vi "Get_Coeff_Fr_String.vi"(4 "String Name":string, 5 "Take New Data?":bool, 6 "Prefix":string, 7 "Show Dialog?":bool=TRUE, 8 "Sub String":string, 9 "Inst type":T1=enum."Raw voltage", 10 "Whole String":string) -> (0 "Coefficients Found?":bool, 2 "Calib Constants":dbl[](array[numeric]))   [LabVIEW 2014]
uses:
  Controls/Pressure_Units.ctl
  Controls/Inst_type.ctl
panel:
  in  "Pressure Units":T2
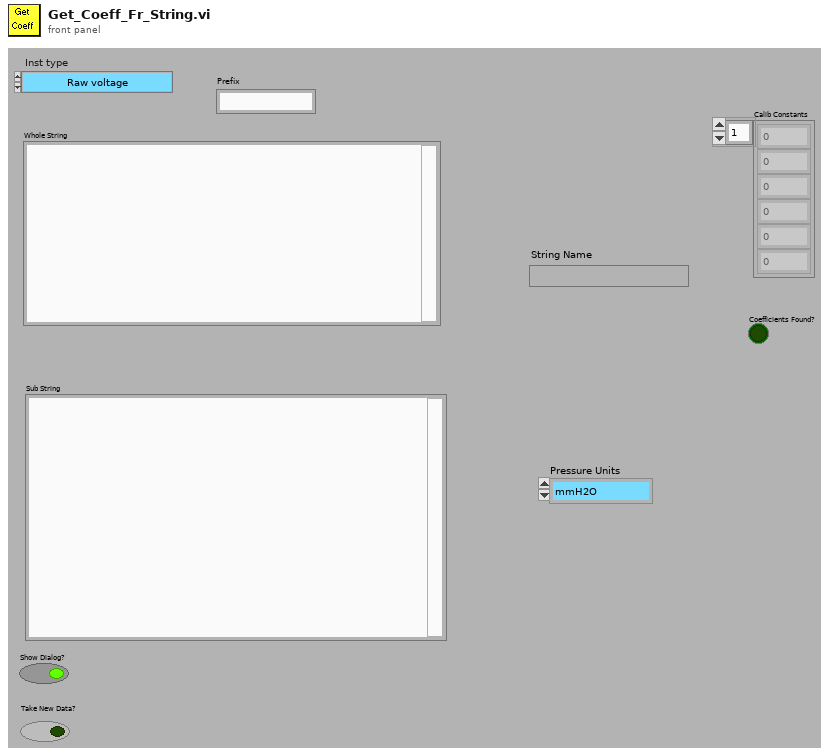
[diagram p1: front panel]
types:
  T1 = typedef "Inst_type.ctl" = enum16{"Propeller anemometer", "Raw voltage", "Pressure Transducer", "Pitot-static tube", "Preston tube", "Hot wire", "Cross wire 1", "Cross wire 2", "Generic Linear", "Generic Polynomial", "Generic BackPoly", "Fast FID", "Thermocouple", "Cold wire", "Pulsed Wire", "LDA Vel", "LDA Tran time", "LDA Arr time", "Microphone"}
  T2 = typedef "Pressure_Units.ctl" = enum16{"mmH2O", "mmHg", "Pa (N/m^2)", "mbar", "bar"}
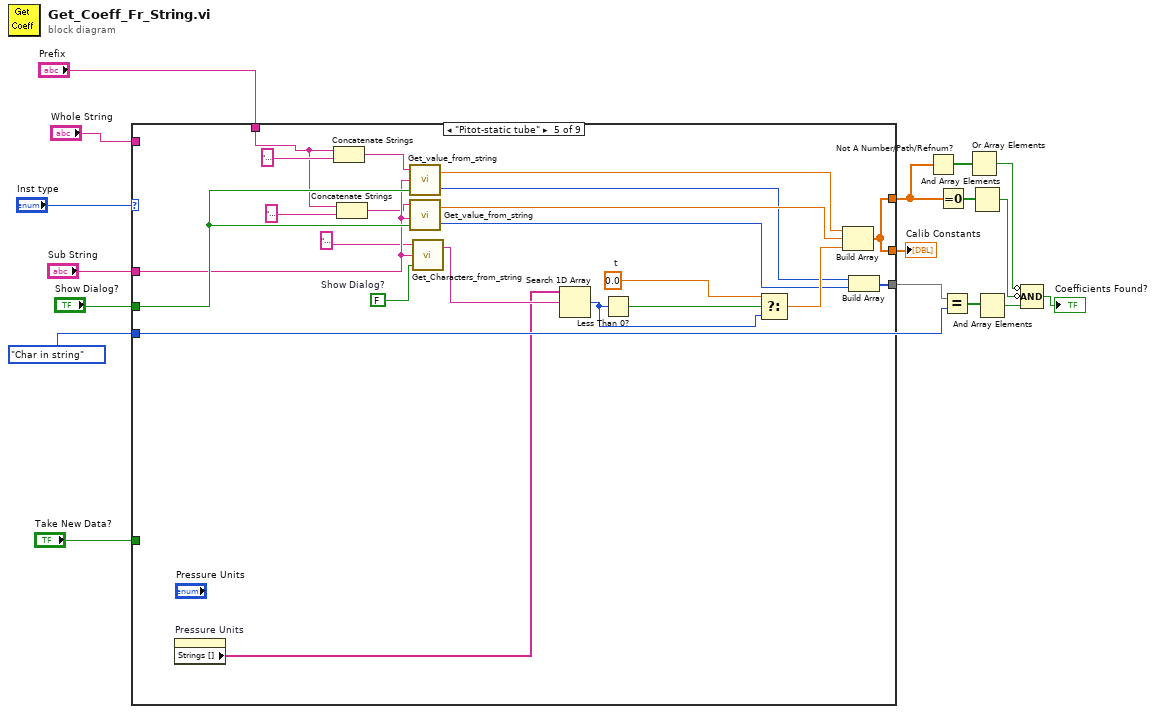
[diagram p0: block diagram]
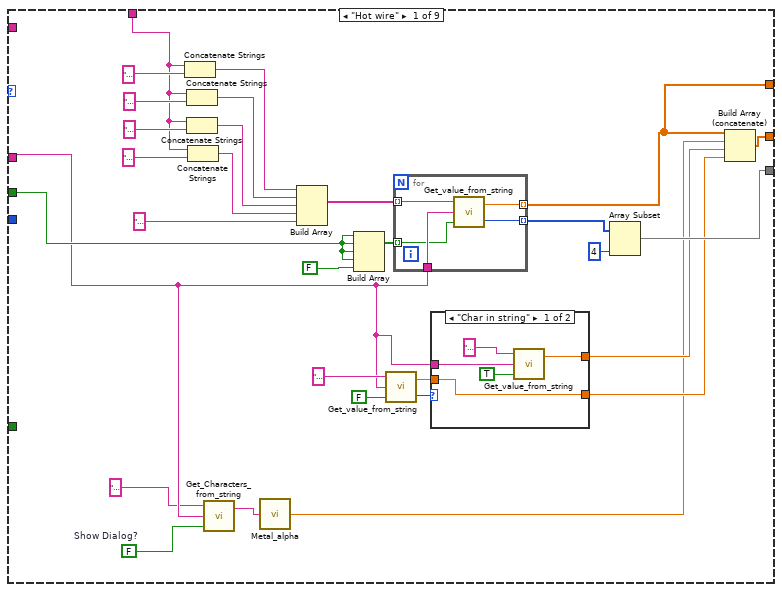
[diagram p2: hidden frame]
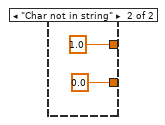
[diagram p3: hidden frame]
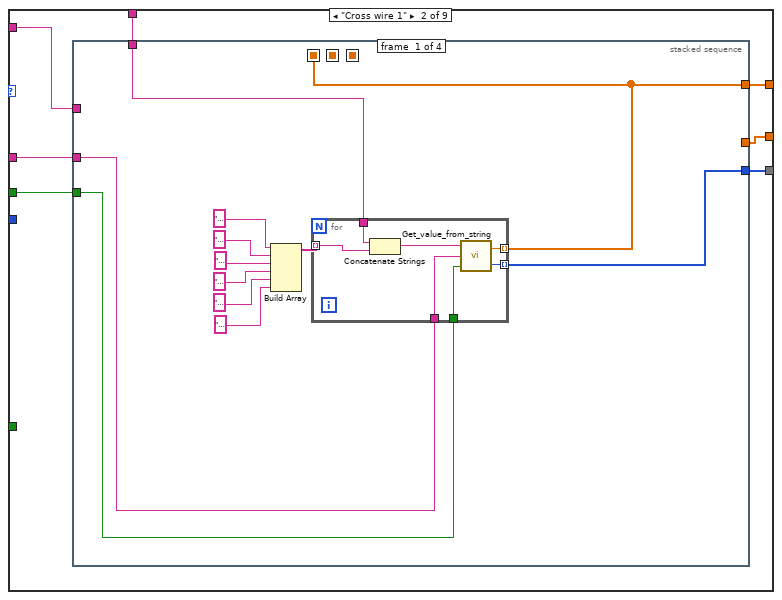
[diagram p4: hidden frame]
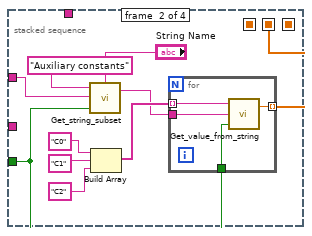
[diagram p5: hidden frame]
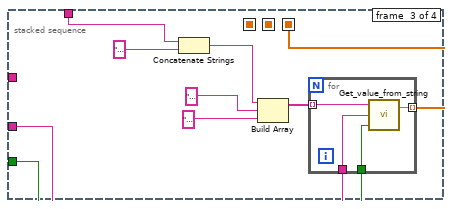
[diagram p6: hidden frame]
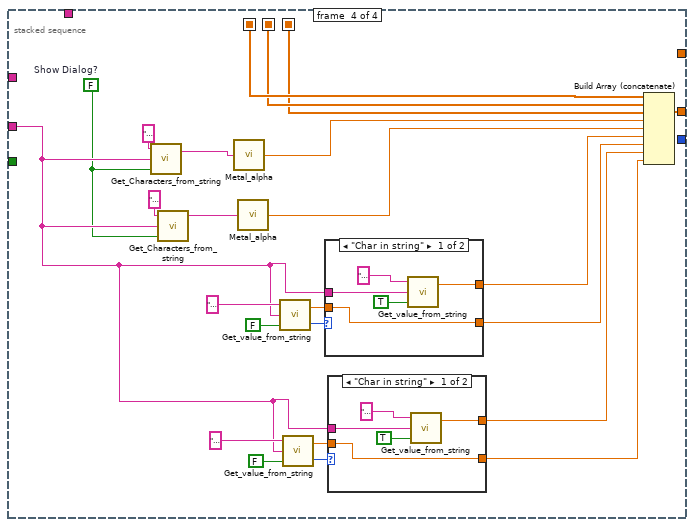
[diagram p7: hidden frame]
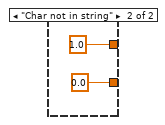
[diagram p8: hidden frame]
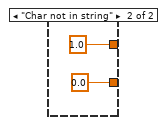
[diagram p9: hidden frame]
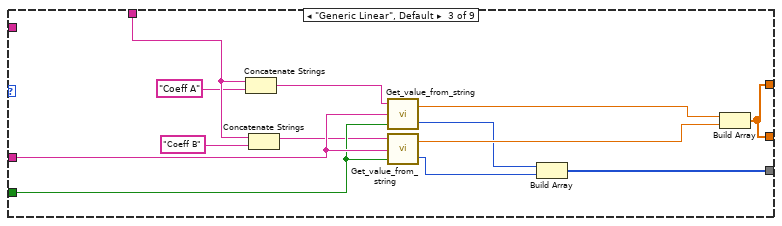
[diagram p10: hidden frame]
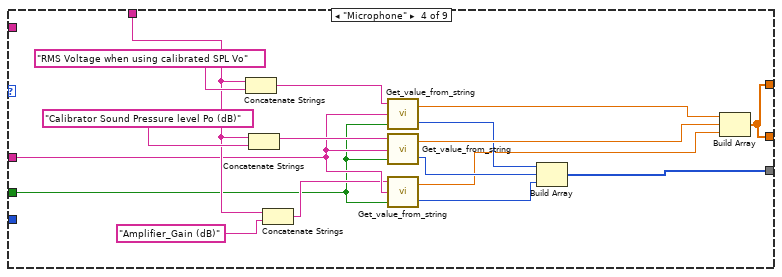
[diagram p11: hidden frame]
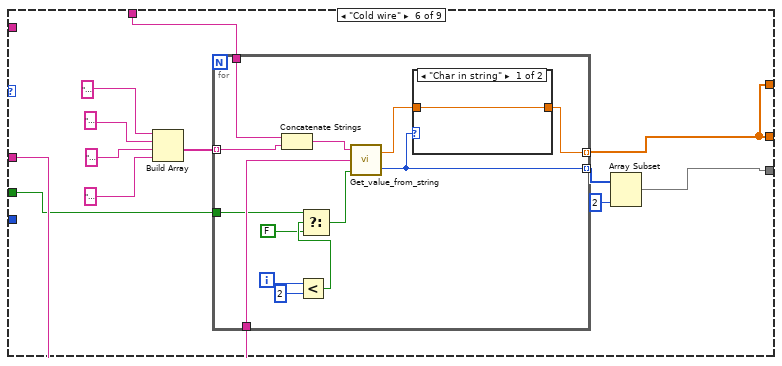
[diagram p12: hidden frame]
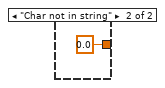
[diagram p13: hidden frame]
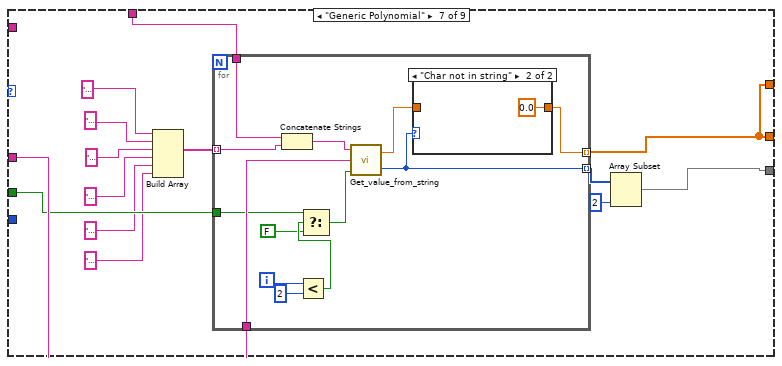
[diagram p14: hidden frame]
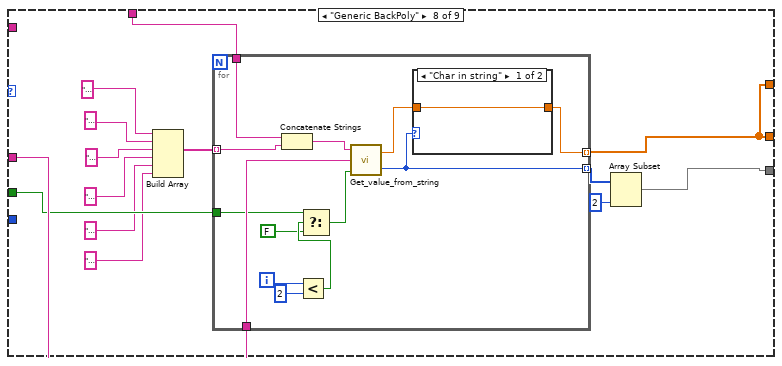
[diagram p16: hidden frame]
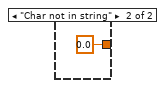
[diagram p17: hidden frame]
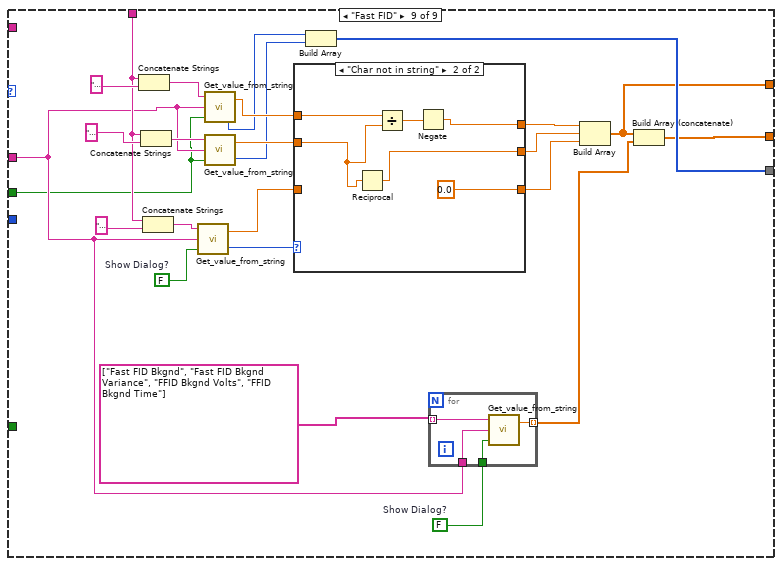
[diagram p18: hidden frame]
diagram:
  w8 = enum16{"Char in string", "Char not in string"}."Char in string" ("Status")
  n1 = case shown="\"Pitot-static tube\"" "Inst type" {
    tunnel: [w47 w66 w151 w171 w181 w202 w231 w260 w288] -> w14
    tunnel: "Sub String" -> [w25 w64 w161 w169 w198 w208 w237 w266 w302]
    tunnel: "Whole String" -> [_ w65 _ _ _ _ _ _ _]
    tunnel: "Show Dialog?" -> [w29 w63 w160 w167 w199 w206 w235 w264 w291]
    tunnel: "Prefix" -> [w37 w62 w159 w170 w184 w207 w236 w265 w305]
    tunnel: "Take New Data?" -> [_ _ _ _ _ _ _ _ _]
    tunnel: [w30 w61 w152 w172 w187 w203 w232 w261 w292] -> w10
    tunnel: w8 -> [_ _ _ _ _ _ _ _ _]
    tunnel: [w21 w60 w151 w171 w181 w202 w231 w260 w287] -> w3
    frame "Hot wire" {
      w44 = FALSE  # Show Dialog?
      n2 = Concatenate Strings(w37, "Coeff A") -> (w33:string)
      n3 = Concatenate Strings(w37, "Coeff B") -> (w34:string)
      n4 = Concatenate Strings(w37, "Coeff n") -> (w35:string)
      n5 = Concatenate Strings(w37, "Calib temp") -> (w36:string)
      n6 = call "Get_Characters_from_string.vi"("Show Dialog?"=w44, "Input string"=w25, "Variable name"="Metal_Type 1") -> ("Value"=w19:string)  [unwired: 1 out]
      n7 = call "Metal_alpha.vi"("Metal_Type"=w19) -> ("alpha (/K)"=w18:dbl)
      n8 = Build Array(w33, w34, w35, w36, "Overheat ratio 1") -> (w45:string[])
      n9 = Build Array(w29, w29, w29, w29, FALSE ("Input Element")) -> (w42:bool[])
      n10 = call "Get_value_from_string.vi"("Show Dialog?"=FALSE, "Input string"=w25, "Variable name"="Offset Voltage 1") -> ("Status"=w26:enum16{"Char in string", "Char not in string"}, "Value"=w23:dbl)
      n11 = for {
        tunnel: w45 -> [w59] mode=indexing
        tunnel: w25 -> [w58]
        tunnel: [w57] -> w21 mode=indexing
        tunnel: w42 -> [w56] mode=indexing
        tunnel: [w55] -> w32 mode=indexing
        n12 = call "Get_value_from_string.vi"("Show Dialog?"=w56, "Input string"=w58, "Variable name"=w59) -> ("Status"=w55:enum16{"Char in string", "Char not in string"}, "Value"=w57:dbl)
      }
      n13 = case shown="\"Char in string\"" w26 {
        tunnel: w25 -> [w52 _]
        tunnel: [w49 1.0 ("Value")] -> w24
        tunnel: w23 -> [w48 _]
        tunnel: [w48 0.0 ("Value")] -> w22
        frame "Char in string" {
          n14 = call "Get_value_from_string.vi"("Show Dialog?"=TRUE, "Input string"=w52, "Variable name"="Gain 1") -> ("Value"=w49:dbl)  [unwired: 1 out]
        }
        frame "Char not in string" {
        }
      }
      n15 = Array Subset(array=w32, length=4) -> (w30:enum16{"Char in string", "Char not in string"}[])  [unwired: 1 in]
      n16 = Build Array (concatenate)(w21, w18, w24, w22) -> (w47:dbl[])
    }
    frame "Cross wire 1" {
      n17 = stacked-sequence {
        seq-local: [w67 _ _ _] -> [_ _ _ w133]
        seq-local: [_ w88 _ _] -> [_ _ _ w132]
        seq-local: [_ _ w105 _] -> [_ _ _ w131]
        tunnel: [_ _ _ w136] -> w66
        tunnel: w65 -> [_ w94 _ _]
        tunnel: w64 -> [w71 _ w107 w122]
        tunnel: w63 -> [w70 w87 w106 _]
        tunnel: w62 -> [w69 _ w100 _]
        tunnel: [w68 _ _ _] -> w61
        tunnel: [w67 _ _ _] -> w60
        frame #0 {
          n18 = Build Array("Coeff A1", "Coeff B1", "Coeff n1", "Coeff A2", "Coeff B2", "Coeff n2") -> (w72:string[])
          n19 = for {
            tunnel: w72 -> [w82] mode=indexing
            tunnel: w71 -> [w85]
            tunnel: [w84] -> w67 mode=indexing
            tunnel: w70 -> [w83]
            tunnel: w69 -> [w80]
            tunnel: [w79] -> w68 mode=indexing
            n20 = Concatenate Strings(w80, w82) -> (w81:string)
            n21 = call "Get_value_from_string.vi"("Show Dialog?"=w83, "Input string"=w85, "Variable name"=w81) -> ("Status"=w79:enum16{"Char in string", "Char not in string"}, "Value"=w84:dbl)
          }
        }
        frame #1 {
          n22 = call "Get_string_subset.vi"("String Name"="String Name", "Show Dialog?"=w87, "String to split"=w94, "File Label"="Auxiliary constants") -> ("Output string"=w89:string)  [unwired: 1 out]
          n23 = Build Array("C0", "C1", "C2") -> (w90:string[])
          n24 = for {
            tunnel: w90 -> [w99] mode=indexing
            tunnel: [w98] -> w88 mode=indexing
            tunnel: w87 -> [w97]
            tunnel: w89 -> [w96]
            n25 = call "Get_value_from_string.vi"("Show Dialog?"=w97, "Input string"=w96, "Variable name"=w99) -> ("Value"=w98:dbl)  [unwired: 1 out]
          }
        }
        frame #2 {
          n26 = Concatenate Strings(w100, "Calib temp") -> (w101:string)
          n27 = Build Array(w101, "Overheat ratio 1", "Overheat ratio 2") -> (w108:string[])
          n28 = for {
            tunnel: w108 -> [w112] mode=indexing
            tunnel: w107 -> [w111]
            tunnel: [w110] -> w105 mode=indexing
            tunnel: w106 -> [w109]
            n29 = call "Get_value_from_string.vi"("Show Dialog?"=w109, "Input string"=w111, "Variable name"=w112) -> ("Value"=w110:dbl)  [unwired: 1 out]
          }
        }
        frame #3 {
          w113 = FALSE  # Show Dialog?
          n30 = call "Get_Characters_from_string.vi"("Show Dialog?"=w113, "Input string"=w122, "Variable name"="Metal_Type 1") -> ("Value"=w116:string)  [unwired: 1 out]
          n31 = call "Get_Characters_from_string.vi"("Show Dialog?"=w113, "Input string"=w122, "Variable name"="Metal_Type 2") -> ("Value"=w117:string)  [unwired: 1 out]
          n32 = call "Metal_alpha.vi"("Metal_Type"=w116) -> ("alpha (/K)"=w115:dbl)
          n33 = call "Metal_alpha.vi"("Metal_Type"=w117) -> ("alpha (/K)"=w114:dbl)
          n34 = call "Get_value_from_string.vi"("Show Dialog?"=FALSE, "Input string"=w122, "Variable name"="Offset Voltage 1") -> ("Status"=w128:enum16{"Char in string", "Char not in string"}, "Value"=w127:dbl)
          n35 = call "Get_value_from_string.vi"("Show Dialog?"=FALSE, "Input string"=w122, "Variable name"="Offset Voltage 2") -> ("Status"=w125:enum16{"Char in string", "Char not in string"}, "Value"=w126:dbl)
          n36 = case shown="\"Char in string\"" w128 {
            tunnel: w122 -> [w148 _]
            tunnel: [w145 1.0 ("Value")] -> w121
            tunnel: w127 -> [w144 _]
            tunnel: [w144 0.0 ("Value")] -> w120
            frame "Char in string" {
              n37 = call "Get_value_from_string.vi"("Show Dialog?"=TRUE, "Input string"=w148, "Variable name"="Gain 1") -> ("Value"=w145:dbl)  [unwired: 1 out]
            }
            frame "Char not in string" {
            }
          }
          n38 = case shown="\"Char in string\"" w125 {
            tunnel: w122 -> [w141 _]
            tunnel: [w138 1.0 ("Value")] -> w118
            tunnel: w126 -> [w137 _]
            tunnel: [w137 0.0 ("Value")] -> w119
            frame "Char in string" {
              n39 = call "Get_value_from_string.vi"("Show Dialog?"=TRUE, "Input string"=w141, "Variable name"="Gain 2") -> ("Value"=w138:dbl)  [unwired: 1 out]
            }
            frame "Char not in string" {
            }
          }
          n40 = Build Array (concatenate)(w133, w132, w131, w115, w114, w121, w120, w118, w119) -> (w136:dbl[])
        }
      }
    }
    frame "Generic Linear", Default {
      n41 = Concatenate Strings(w159, "Coeff A") -> (w155:string)
      n42 = Concatenate Strings(w159, "Coeff B") -> (w156:string)
      n43 = call "Get_value_from_string.vi"("Show Dialog?"=w160, "Input string"=w161, "Variable name"=w155) -> ("Status"=w154:enum16{"Char in string", "Char not in string"}, "Value"=w162:dbl)
      n44 = call "Get_value_from_string.vi"("Show Dialog?"=w160, "Input string"=w161, "Variable name"=w156) -> ("Status"=w153:enum16{"Char in string", "Char not in string"}, "Value"=w163:dbl)
      n45 = Build Array(w154, w153) -> (w152:enum16{"Char in string", "Char not in string"}[])
      n46 = Build Array(w162, w163) -> (w151:dbl[])
    }
    frame "Microphone" {
      n47 = Concatenate Strings(w170, "RMS Voltage when using calibrated SPL Vo") -> (w175:string)
      n48 = Concatenate Strings(w170, "Calibrator Sound Pressure level Po (dB)") -> (w176:string)
      n49 = Concatenate Strings(w170, "Amplifier_Gain (dB)") -> (w168:string)
      n50 = call "Get_value_from_string.vi"("Show Dialog?"=w167, "Input string"=w169, "Variable name"=w175) -> ("Status"=w174:enum16{"Char in string", "Char not in string"}, "Value"=w179:dbl)
      n51 = call "Get_value_from_string.vi"("Show Dialog?"=w167, "Input string"=w169, "Variable name"=w176) -> ("Status"=w173:enum16{"Char in string", "Char not in string"}, "Value"=w180:dbl)
      n52 = call "Get_value_from_string.vi"("Show Dialog?"=w167, "Input string"=w169, "Variable name"=w168) -> ("Status"=w166:enum16{"Char in string", "Char not in string"}, "Value"=w165:dbl)
      n53 = Build Array(w174, w173, w166) -> (w172:enum16{"Char in string", "Char not in string"}[])
      n54 = Build Array(w179, w180, w165) -> (w171:dbl[])
    }
    frame "Pitot-static tube" {
      w192 = 0.0  # t
      w196 = FALSE  # Show Dialog?
      n55 = property on="Pressure Units" class="Enum (strict)"() -> ("Strings []"=w190:string[])  [unwired: 2 in, 2 out]
      n56 = Concatenate Strings(w184, "Coeff A") -> (w183:string)
      n57 = Concatenate Strings(w184, "Coeff B") -> (w182:string)
      n58 = call "Get_value_from_string.vi"("Show Dialog?"=w199, "Input string"=w198, "Variable name"=w183) -> ("Status"=w189:enum16{"Char in string", "Char not in string"}, "Value"=w200:dbl)
      n59 = call "Get_value_from_string.vi"("Show Dialog?"=w199, "Input string"=w198, "Variable name"=w182) -> ("Status"=w188:enum16{"Char in string", "Char not in string"}, "Value"=w201:dbl)
      n60 = call "Get_Characters_from_string.vi"("Show Dialog?"=w196, "Input string"=w198, "Variable name"="Pressure_Transducer_Units") -> ("Value"=w195:string)  [unwired: 1 out]
      n61 = Search 1D Array(1D array=w190, element=w195) -> (index of element=w193:i32)  [unwired: 1 out]
      n62 = Less Than 0?(x=w193) -> (x < 0?=w194:bool)
      n63 = Select(t=w192, s=w194, f=w193) -> (s? t:f=w191:dbl)
      n64 = Build Array(w200, w201, w191) -> (w181:dbl[])
      n65 = Build Array(w189, w188) -> (w187:enum16{"Char in string", "Char not in string"}[])
    }
    frame "Cold wire" {
      n66 = Build Array("Coeff A", "Coeff B", "Coeff C", "Coeff D") -> (w209:string[])
      n67 = for {
        tunnel: w209 -> [w225] mode=indexing
        tunnel: w208 -> [w226]
        tunnel: [w215] -> w202 mode=indexing
        tunnel: w207 -> [w224]
        tunnel: [w216] -> w204 mode=indexing
        tunnel: w206 -> [w219]
        i -> [w222]
        n68 = Concatenate Strings(w224, w225) -> (w223:string)
        n69 = Less?(x=w222, y=2) -> (x < y?=w220:bool)
        n70 = Select(t=w219, s=w220, f=FALSE) -> (s? t:f=w217:bool)
        n71 = call "Get_value_from_string.vi"("Show Dialog?"=w217, "Input string"=w226, "Variable name"=w223) -> ("Status"=w216:enum16{"Char in string", "Char not in string"}, "Value"=w214:dbl)
        n72 = case shown="\"Char in string\"" w216 {
          tunnel: [w227 0.0 ("Value")] -> w215
          tunnel: w214 -> [w227 _]
          frame "Char in string" {
          }
          frame "Char not in string" {
          }
        }
      }
      n73 = Array Subset(array=w204, length=2) -> (w203:enum16{"Char in string", "Char not in string"}[])  [unwired: 1 in]
    }
    frame "Generic Polynomial" {
      n74 = Build Array("Coeff A", "Coeff B", "Coeff C", "Coeff D", "Coeff E", "Coeff F") -> (w238:string[])
      n75 = for {
        tunnel: w238 -> [w254] mode=indexing
        tunnel: w237 -> [w255]
        tunnel: [w244] -> w231 mode=indexing
        tunnel: w236 -> [w253]
        tunnel: [w245] -> w233 mode=indexing
        tunnel: w235 -> [w248]
        i -> [w251]
        n76 = Concatenate Strings(w253, w254) -> (w252:string)
        n77 = Less?(x=w251, y=2) -> (x < y?=w249:bool)
        n78 = Select(t=w248, s=w249, f=FALSE) -> (s? t:f=w246:bool)
        n79 = call "Get_value_from_string.vi"("Show Dialog?"=w246, "Input string"=w255, "Variable name"=w252) -> ("Status"=w245:enum16{"Char in string", "Char not in string"}, "Value"=w243:dbl)
        n80 = case shown="\"Char not in string\"" w245 {
          tunnel: [w256 0.0 ("Value")] -> w244
          tunnel: w243 -> [w256 _]
          frame "Char in string" {
          }
          frame "Char not in string" {
          }
        }
      }
      n81 = Array Subset(array=w233, length=2) -> (w232:enum16{"Char in string", "Char not in string"}[])  [unwired: 1 in]
    }
    frame "Generic BackPoly" {
      n82 = Build Array("Coeff A", "Coeff B", "Coeff C", "Coeff D", "Coeff E", "Coeff F") -> (w267:string[])
      n83 = for {
        tunnel: w267 -> [w283] mode=indexing
        tunnel: w266 -> [w284]
        tunnel: [w273] -> w260 mode=indexing
        tunnel: w265 -> [w282]
        tunnel: [w274] -> w262 mode=indexing
        tunnel: w264 -> [w277]
        i -> [w280]
        n84 = Concatenate Strings(w282, w283) -> (w281:string)
        n85 = Less?(x=w280, y=2) -> (x < y?=w278:bool)
        n86 = Select(t=w277, s=w278, f=FALSE) -> (s? t:f=w275:bool)
        n87 = call "Get_value_from_string.vi"("Show Dialog?"=w275, "Input string"=w284, "Variable name"=w281) -> ("Status"=w274:enum16{"Char in string", "Char not in string"}, "Value"=w272:dbl)
        n88 = case shown="\"Char in string\"" w274 {
          tunnel: [w285 0.0 ("Value")] -> w273
          tunnel: w272 -> [w285 _]
          frame "Char in string" {
          }
          frame "Char not in string" {
          }
        }
      }
      n89 = Array Subset(array=w262, length=2) -> (w261:enum16{"Char in string", "Char not in string"}[])  [unwired: 1 in]
    }
    frame "Fast FID" {
      w290 = FALSE  # Show Dialog?
      w311 = FALSE  # Show Dialog?
      n90 = Concatenate Strings(w305, "Coeff A") -> (w308:string)
      n91 = Concatenate Strings(w305, "Coeff B") -> (w306:string)
      n92 = Concatenate Strings(w305, "Coeff C") -> (w303:string)
      n93 = call "Get_value_from_string.vi"("Show Dialog?"=w311, "Input string"=w302, "Variable name"=w303) -> ("Status"=w310:enum16{"Char in string", "Char not in string"}, "Value"=w295:dbl)
      n94 = call "Get_value_from_string.vi"("Show Dialog?"=w291, "Input string"=w302, "Variable name"=w308) -> ("Status"=w294:enum16{"Char in string", "Char not in string"}, "Value"=w301:dbl)
      n95 = call "Get_value_from_string.vi"("Show Dialog?"=w291, "Input string"=w302, "Variable name"=w306) -> ("Status"=w293:enum16{"Char in string", "Char not in string"}, "Value"=w300:dbl)
      n96 = case shown="\"Char not in string\"" w310 {
        tunnel: w301 -> [w318 w323]
        tunnel: w300 -> [w317 w322]
        tunnel: [w318 w321] -> w299
        tunnel: [w317 w320] -> w298
        tunnel: [w316 0.0 ("new element/subarray")] -> w297
        tunnel: w295 -> [w316 _]
        frame "Char in string" {
        }
        frame "Char not in string" {
          n97 = Reciprocal(x=w322) -> (1/x=w320:dbl)
          n98 = Divide(x=w323, y=w322) -> (x/y=w324:dbl)
          n99 = Negate(x=w324) -> (-x=w321:dbl)
        }
      }
      n100 = Build Array(w294, w293) -> (w292:enum16{"Char in string", "Char not in string"}[])
      n101 = for {
        tunnel: string[] ["Fast FID Bkgnd", "Fast FID Bkgnd Variance", "FFID Bkgnd Volts", "FFID Bkgnd Time"] ("appended array") -> [w315] mode=indexing
        tunnel: w302 -> [w314]
        tunnel: [w313] -> w289 mode=indexing
        tunnel: w290 -> [w312]
        n102 = call "Get_value_from_string.vi"("Show Dialog?"=w312, "Input string"=w314, "Variable name"=w315) -> ("Value"=w313:dbl)  [unwired: 1 out]
      }
      n103 = Build Array(w299, w298, w297) -> (w287:dbl[])
      n104 = Build Array (concatenate)(w287, w289) -> (w288:dbl[])
    }
  }
  "Calib Constants" <- w14
  n105 = Not A Number/Path/Refnum?(number/path/refnum=w3) -> (NaN/Path/Refnum?=w2:bool[])
  n106 = Equal To 0?(x=w3) -> (x = 0?=w4:bool[])
  n107 = Equal?(x=w10, y=w8) -> (x = y?=w9:bool[])
  n108 = Or Array Elements(Boolean array=w2) -> (logical OR=w1:bool)
  n109 = And Array Elements(Boolean array=w4) -> (logical AND=w5:bool)
  n110 = And Array Elements(Boolean array=w9) -> (logical AND=w7:bool)
  n111 = Compound Arithmetic op=AND(invert w1, invert w5, w7) -> (→"Coefficients Found?":bool)
